vi "Sequencing Engine.vi"() -> ()   [LabVIEW 2014]
uses:
  Initialization Scripting/Initialization and IO Node Scripting.lvlib
panel:
  in  "Path to Test VI to Place (IO Nodes and SPI Engine Placed on Block Diagram)":path=path "C:/Users/mpool/Desktop/test/TestVI.vi"
  in  "Path to Test Project":path=path "C:/Users/lvadmin/Desktop/Scripting/Test/Test.lvproj"
  in  "Error In":errorcluster
  in  "Enable":bool[](array[boolean])=[TRUE, FALSE, FALSE, FALSE, TRUE, FALSE, TRUE, TRUE, TRUE]
  in  "List of Enable Lines":string[](array[string])=["sbRIO-9651 Socket\\PMOD1_Pin3_enable", "sbRIO-9651 Socket\\PMOD1_Pin4_enable"]
  in  "List of IO Names":string[](array[string])=["Port0/DIO0", "Port0/DIO5", "Port0/DIO6"]
  out "Error Out":errorcluster
  in  "Number of SPI Devices on Bus":i32=2
  in  "Destination Path":path=path "C:/Users/kvemishe/Downloads/TestScript"
  in  "Golden Template Source Path":path=path "C:/Users/kvemishe/Desktop/IONode"
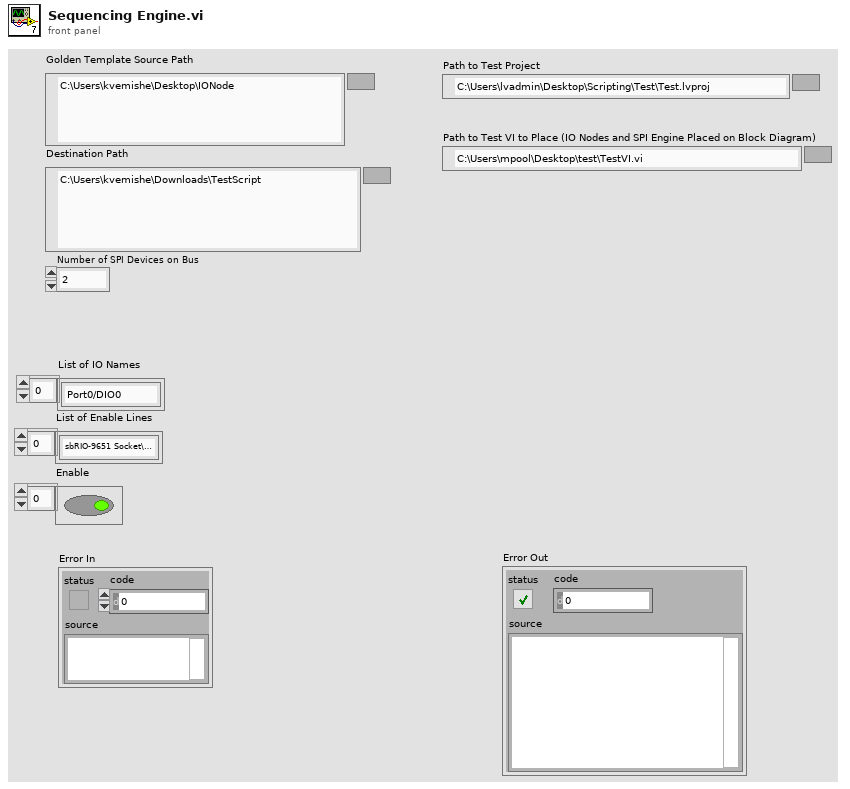
[diagram p1: front panel]
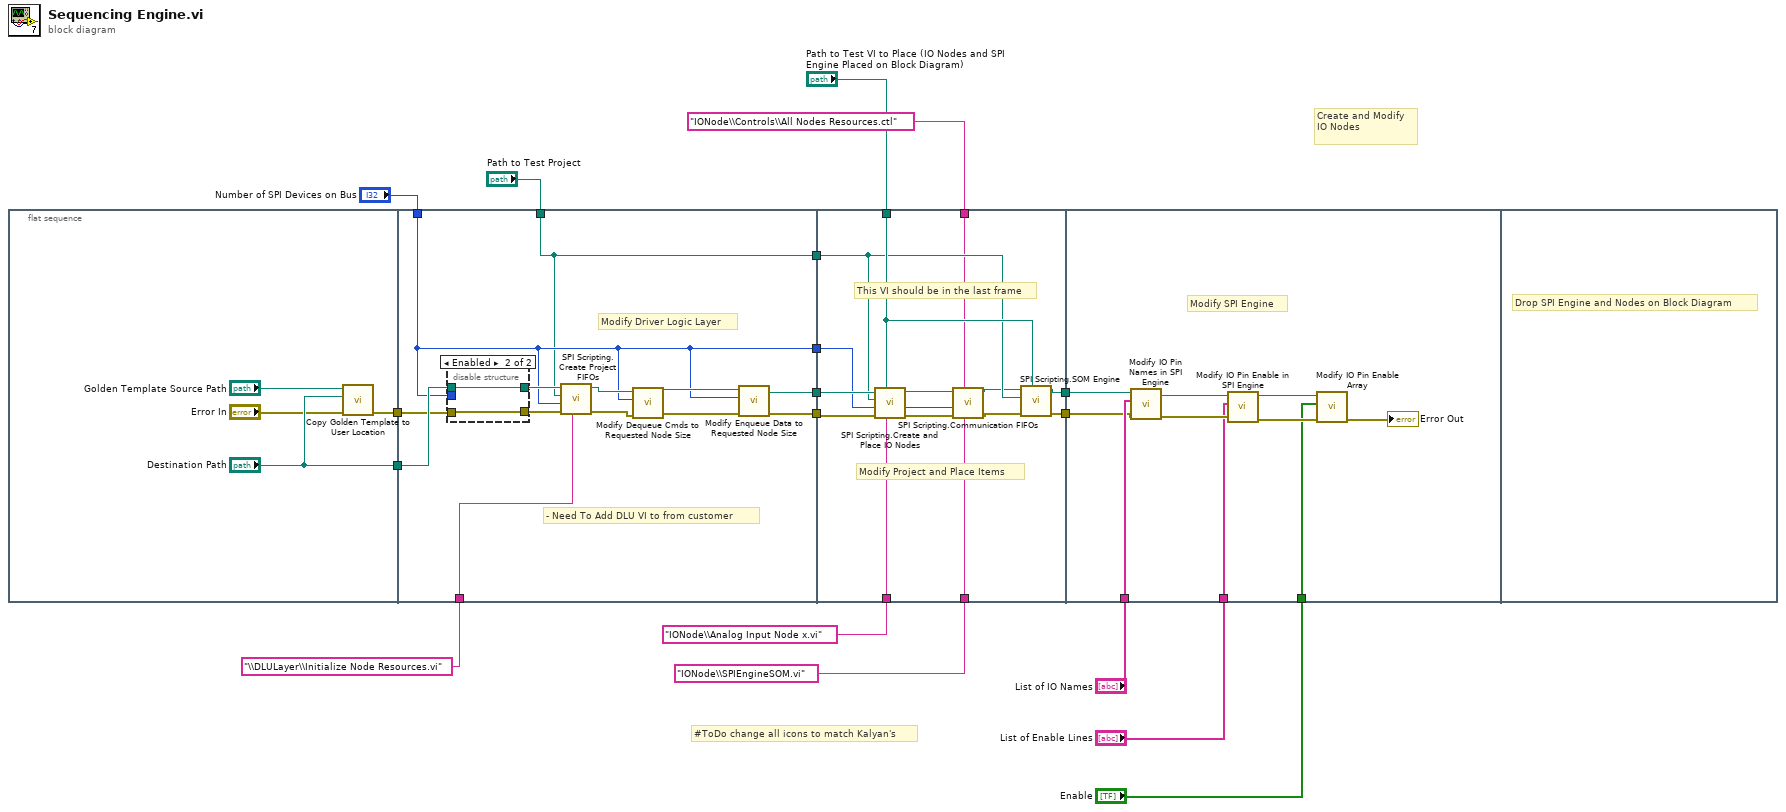
[diagram p0: block diagram]
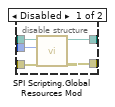
[diagram p2: hidden frame]
diagram:
  # "#ToDo change all icons to match Kalyan's"
  # "Create and Modify IO Nodes"
  n1 = flat-sequence {
    tunnel: ["Destination Path"] -> w17
    tunnel: [w20] -> w16
    tunnel: w16 -> [w30]
    tunnel: w17 -> [w31]
    tunnel: "Number of SPI Devices on Bus" -> [w25]
    tunnel: [w33] -> w15
    tunnel: [w32] -> w12
    tunnel: [w25] -> w8
    tunnel: "Path to Test Project" -> [w24]
    tunnel: [w24] -> w5
    tunnel: "\\DLULayer\\Initialize Node Resources.vi" ("Path of Initialization VI") -> [w23]
    tunnel: w15 -> [w55]
    tunnel: [w57] -> w14
    tunnel: w12 -> [w54]
    tunnel: [w56] -> w9
    tunnel: w8 -> [w52]
    tunnel: "Path to Test VI to Place (IO Nodes and SPI Engine Placed on Block Diagram)" -> [w53]
    tunnel: w5 -> [w51]
    tunnel: "IONode\\Controls\\All Nodes Resources.ctl" ("Path to All Nodes Resources") -> [w48]
    tunnel: "IONode\\Analog Input Node x.vi" ("Path to SOM Engine") -> [w50]
    tunnel: "IONode\\SPIEngineSOM.vi" ("Path to SOM Engine") -> [w43]
    tunnel: w14 -> [w67]
    tunnel: "List of IO Names" -> [w66]
    tunnel: "List of Enable Lines" -> [w62]
    tunnel: "Enable" -> [w58]
    tunnel: w9 -> [w65]
    frame #0 {
      n2 = call "Copy Golden Template to User Location.vi"("Error In"="Error In", "Current Engine Path"="Destination Path", "Golden Template Path"="Golden Template Source Path") -> ("error out"=w20:errorcluster)  [unwired: 8 in]
    }
    frame #1 {
      # "- Need To Add DLU VI to from customer"
      # "Modify Driver Logic Layer"
      n3 = disable-structure shown="Enabled" {
        disable-tunnel: w31 -> [w40 w42]
        disable-tunnel: [w39 w42] -> w28
        disable-tunnel: w30 -> [w38 w41]
        disable-tunnel: [w37 w41] -> w29
        disable-tunnel: w25 -> [w36 _]
        frame Disabled {
          n4 = call "SPI Scripting.Global Resources Mod.vi"("error in"=w38, "Number of SPI Devices on Bus"=w36, "Path to IO Node"=w40) -> ("error out"=w37:errorcluster, "Path to IO Node"=w39:path)  [unwired: 6 in, 1 out]
        }
        frame Enabled {
        }
      }
      n5 = call "SPI Scripting.Create Project FIFOs.vi"("Path of Initialization VI"=w23, "error in"=w29, "Number of SPI Devices on Bus"=w25, "Path to Project"=w24, "Path to IO Node"=w28) -> ("error out"=w26:errorcluster, "Path to IO Node"=w27:path)  [unwired: 4 in, 1 out]
      n6 = call "Modify Dequeue Cmds to Requested Node Size.vi"("Error In"=w26, "NumCasesToAdd"=w25, "Source Root Path"=w27) -> ("Error Out"=w34:errorcluster, "Source Root Path Out"=w35:path)  [unwired: 6 in, 1 out]
      n7 = call "Modify Enqueue Data to Requested Node Size.vi"("Error In"=w34, "NumCasesToAdd"=w25, "Source Root Path"=w35) -> ("error out"=w32:errorcluster, "Source Root Path Out"=w33:path)  [unwired: 6 in, 1 out]
    }
    frame #2 {
      # "This VI should be in the last frame"
      # "Modify Project and Place Items"
      n8 = call "SPI Scripting.Create and Place IO Nodes.vi"("Path to Analog Node"=w50, "Path to Place IO Node"=w53, "error in"=w54, "Number of SPI Devices on Bus"=w52, "Path to Project"=w51, "Path to IO Node"=w55) -> ("error out"=w47:errorcluster, "Number of SPI Devices on Bus"=w46:i32, "Path to IO Node"=w49:path)  [unwired: 3 in]
      n9 = call "SPI Scripting.Communication FIFOs.vi"("Path to SOM Engine"=w43, "Path to All Nodes Resources"=w48, "error in"=w47, "Number of SPI Devices on Bus"=w46, "Path to IO Node"=w49) -> ("error out"=w45:errorcluster, "Path to IO Node"=w44:path)  [unwired: 4 in, 1 out]
      n10 = call "SPI Scripting.SOM Engine.vi"("Path to Place SPI Engine"=w53, "error in"=w45, "Path to Project"=w51, "Path to IO Node"=w44) -> ("error out"=w56:errorcluster, "Path to IO Node"=w57:path)  [unwired: 6 in]
    }
    frame #3 {
      # "Modify SPI Engine"
      n11 = call "Modify IO Pin Names in SPI Engine.vi"("Error In"=w65, "List of IO Names"=w66, "Source Root Path"=w67) -> ("Error Out"=w63:errorcluster, "Source Root Path Out"=w64:path)  [unwired: 6 in, 1 out]
      n12 = call "Modify IO Pin Enable in SPI Engine.vi"("Error In"=w63, "List of Enable Lines"=w62, "Source Root Path"=w64) -> ("Error Out"=w60:errorcluster, "Source Root Path Out"=w61:path)  [unwired: 6 in, 1 out]
      n13 = call "Modify IO Pin Enable Array.vi"("Error In"=w60, "Enable"=w58, "Source Root Path"=w61) -> ("Error Out"=→"Error Out":errorcluster)  [unwired: 6 in, 2 out]
    }
    frame #4 {
      # "Drop SPI Engine and Nodes on Block Diagram"
    }
  }
